vi "Registers.vi"   [LabVIEW 2021]
uses:
  <userlib>/SciSDK/SciSDK_Labview.lvlib
types:
  T1 = cluster{"Name":string, "Board Model":string, "Handle":u64}
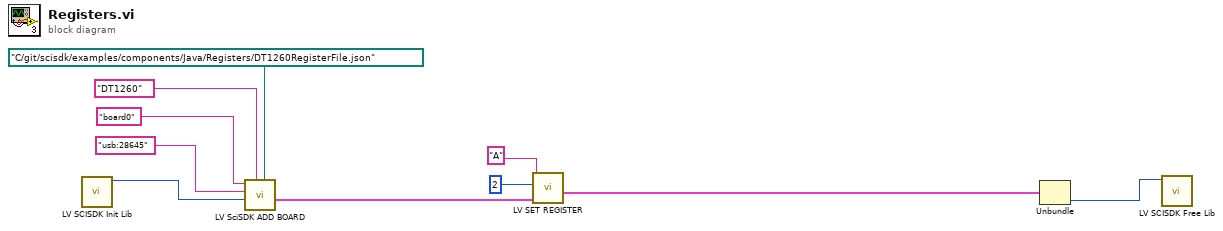
[diagram p0: block diagram]
diagram:
  n1 = call <userlib>:"LV SCISDK Init Lib.vi"() -> ("function return"=w10:u64)  [unwired: 11 in]
  n2 = call <userlib>:"LV SciSDK ADD BOARD.vi"("JsonFile"=path "C:/git/scisdk/examples/components/Java/Registers/DT1260RegisterFile.json", "Board Model"="DT1260", "SciSDK Handle"=w10, "DevicePath"="usb:28645", "Name"="board0") -> ("Board Handle Out"=w4:T1)  [unwired: 4 in, 2 out]
  n3 = call <userlib>:"LV SET REGISTER.vi"("Board Handle In"=w4, "Value"=u32 2, "Name"="A" ("Register Name")) -> ("Board Handle Out"=w1:T1)  [unwired: 6 in, 2 out]
  n4 = Unbundle(w1) -> ("Handle"=w9:u64)  [unwired: 2 out]
  n5 = call <userlib>:"LV SCISDK Free Lib.vi"("handle"=w9) -> ()  [unwired: 9 in, 2 out]
